vi "loadDataToBuffer.vi"(8 "error in (no error)":errorcluster, 11 "SoundAO in":refnum<class "SoundAO.lvclass">) -> (0 "error out":errorcluster, 3 "SoundAO out":refnum<class "SoundAO.lvclass">)   [LabVIEW 2009, in "Hardware.lvlib" / "Channels.lvlib" / "SoundAO.lvclass"]
doc: "Abstract Method.\n\nThis vi, via its implementing classes, loads the analog output data to the buffer of the device."
uses:
  SoundAO.lvclass
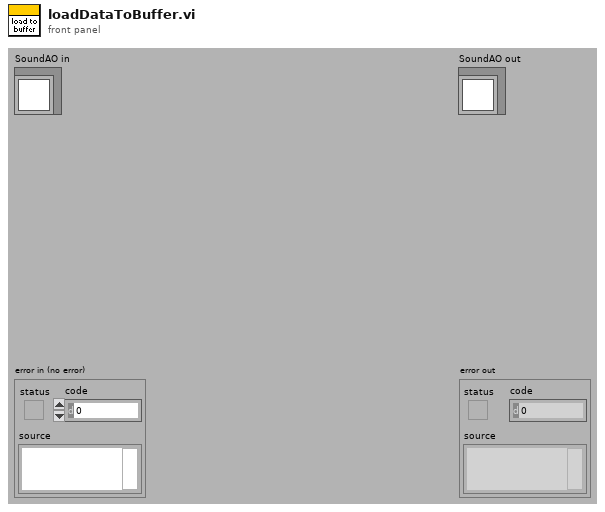
[diagram p1: front panel]
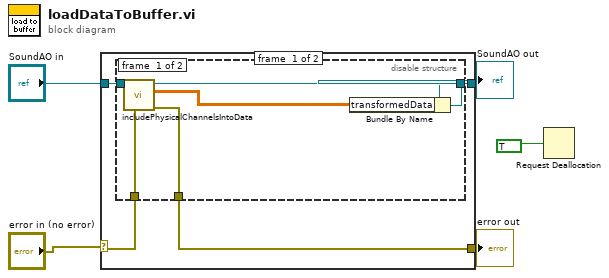
[diagram p0: block diagram]
diagram:
  n1 = case shown="No Error" "error in (no error)" {
    selector: "error in (no error)" -> [w8 w18]
    tunnel: [w7 w19] -> w2
    tunnel: "SoundAO in" -> [w9 w19]
    tunnel: [w6 w18] -> w3
    frame #0 {
      n2 = disable-structure shown="Enabled" {
        disable-tunnel: w9 -> [w15 w17]
        disable-tunnel: w8 -> [w14 w16]
        disable-tunnel: [w11 w17] -> w7
        disable-tunnel: [w10 w16] -> w6
        frame #0 {
          n3 = call "includePhysicalChannelsIntoData.vi"("error in (no error)"=w14, "SoundAO in"=w15) -> ("error out"=w10:errorcluster, "transformedData"=w12:dbl[][], "SoundAO out"=w13:refnum<class "SoundAO.lvclass">)  [unwired: 7 in]
          n4 = Bundle By Name(cluster=w13, "transformedData"=w12) -> (w11:refnum<class "SoundAO.lvclass">)
        }
        frame #1 {
        }
      }
    }
    frame #1 {
    }
  }
  "error out" <- w3
  "SoundAO out" <- w2
  n5 = Request Deallocation(TRUE) -> ()
